vi "Read TestCase map.vi"(8 "error in (no error)":errorcluster, 11 "Test Finder In":refnum<class "Test Finder.lvclass">) -> (0 "error out":errorcluster, 2 "TestCase map":map{string, map{string, path}}(c390), 3 "Test Finder Out":refnum<class "Test Finder.lvclass">)   [LabVIEW 2020, in "Test Finder.lvclass"]
uses:
  Test Finder.lvclass
  Test Finder.lvclass/Test Finder.ctl
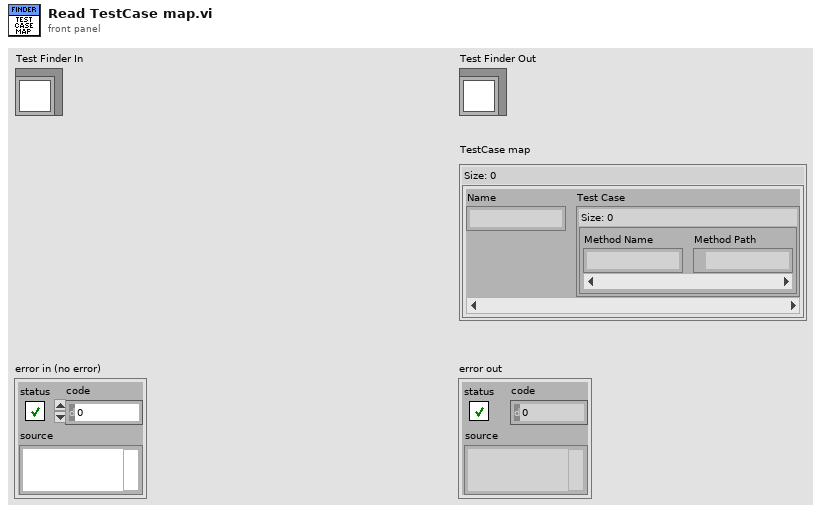
[diagram p1: front panel]
types:
  T1 = map{string, cluster{"Inherited Methods":map{string, path}, "Owned Methods":map{string, path}}}
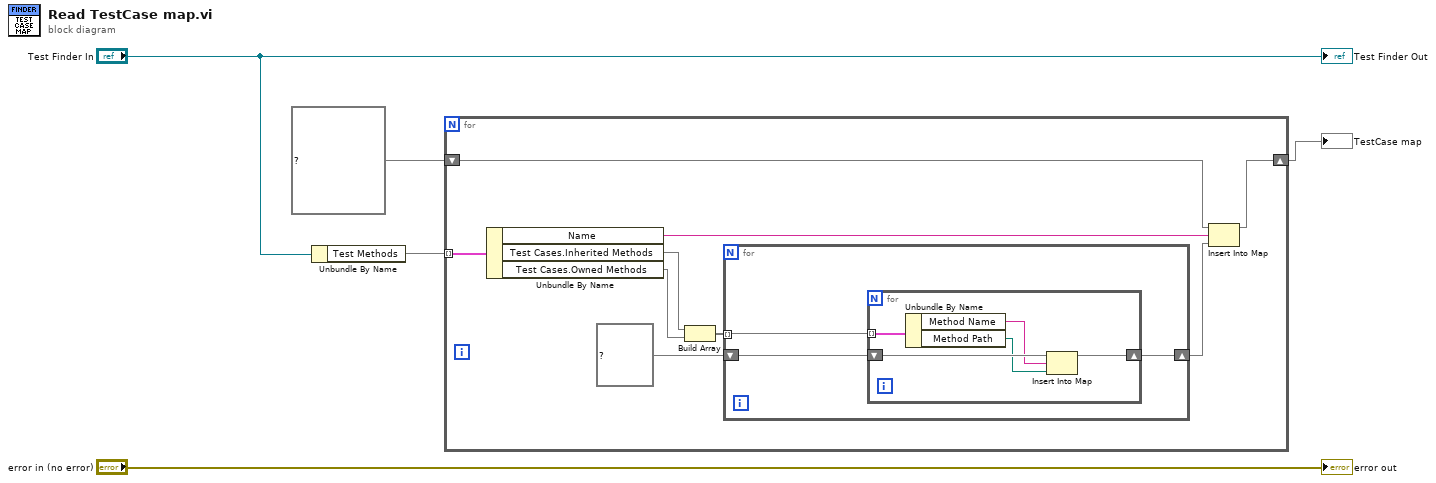
[diagram p0: block diagram]
diagram:
  n1 = Unbundle By Name("Test Finder In") -> ("Test Methods"=w3:T1)
  n2 = for {
    tunnel: w3 -> [w14] mode=indexing
    shift-right: [w10] -> w1
    shift-left: map{string, map{string, path}} {} ("TestCase map") -> [w11]
    n3 = Unbundle By Name(w14) -> ("Name"=w8:string, "Test Cases.Inherited Methods"=w12:map{string, path}, "Test Cases.Owned Methods"=w6:map{string, path})
    n4 = Build Array(w12, w6) -> (w7:map{string, path}[])
    n5 = for {
      tunnel: w7 -> [w15] mode=indexing
      shift-right: [w16] -> w9
      shift-left: map{string, path} {} ("Test Cases.Dynamic Methods") -> [w17]
      n6 = for {
        shift-right: [w21] -> w16
        shift-left: w17 -> [w22]
        tunnel: w15 -> [w20] mode=indexing
        n7 = Unbundle By Name(w20) -> ("Method Name"=w19:string, "Method Path"=w18:path)
        n8 = Insert Into Map(map in=w22, key=w19, value=w18) -> (map out=w21:map{string, path})  [unwired: 2 out]
      }
    }
    n9 = Insert Into Map(map in=w11, key=w8, value=w9) -> (map out=w10:map{string, map{string, path}})  [unwired: 2 out]
  }
  "TestCase map" <- w1
  "error out" <- "error in (no error)"
  "Test Finder Out" <- "Test Finder In"
